vi "Parse qUSG CMD Answer.vi"(0 "Answer To Parse":string, 5 "error in":errorcluster) -> (14 "Array of CommandInfo":T1[](array[typedef]), 19 "error out":errorcluster)   [LabVIEW 2020]
doc: "Parse a SPV? structured answer to a array of parameter sets.\nWill return a warning if some parameters could not be parsed."
uses:
  General command.llb/CommandInfo.ctl
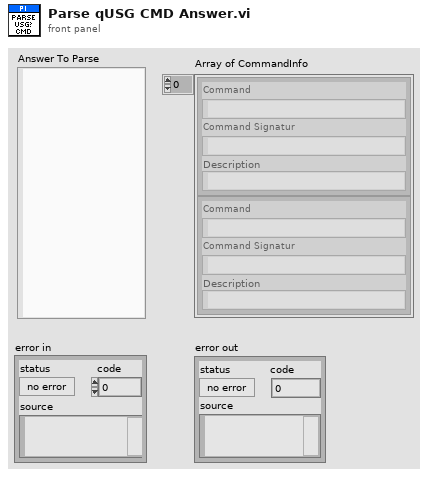
[diagram p1: front panel]
types:
  T1 = typedef "CommandInfo.ctl" = cluster{"Command":string, "Command Signatur":string, "Description":string}
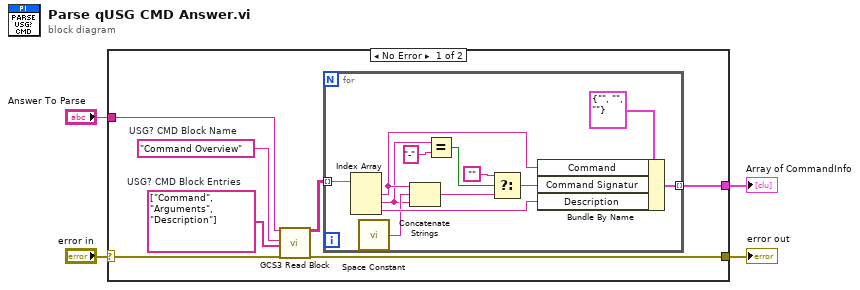
[diagram p0: block diagram]
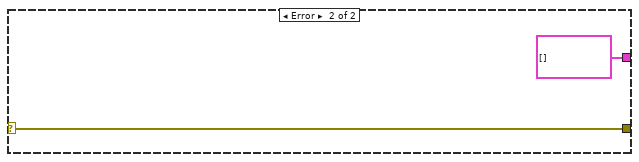
[diagram p2: hidden frame]
diagram:
  n1 = case shown="No Error" "error in" {
    selector: "error in" -> [w10 w25]
    tunnel: "Answer To Parse" -> [w11 _]
    tunnel: [w5 T1[] []] -> w1
    tunnel: [w6 w25] -> w2
    frame No Error {
      w7 = string[] ["Command", "Arguments", "Description"]  # USG? CMD Block Entries
      w8 = "Command Overview"  # USG? CMD Block Name
      n2 = call "GCS3 Read Block.vi"("GCS 3.0 Block to Parse"=w11, "Expected GCS 3.0 Block Name"=w8, "List of expected GCS 3.0 Block Entries"=w7, "error in"=w10) -> ("List of extracted GCS 3.0 Block Entries"=w9:string[][], "error out"=w6:errorcluster)  [unwired: 14 in]
      n3 = for {
        tunnel: w9 -> [w20] mode=indexing
        tunnel: [w21] -> w5 mode=indexing
        n4 = Index Array(array=w20) -> (element #1=w14:string, element #2=w13:string, element #3=w23:string)  [unwired: 3 in]
        n5 = call <vilib>:"Space Constant.vi"() -> ("String"=w15:string)
        n6 = Concatenate Strings(w14, w15, w13) -> (w16:string)
        n7 = Equal?(x=w13, y="-") -> (x = y?=w19:bool)
        n8 = Select(t="", s=w19, f=w16) -> (s? t:f=w12:string)
        n9 = Bundle By Name(cluster=T1 {"Command"="", "Command Signatur"="", "Description"=""} ("CommandInfo"), "Command"=w14, "Command Signatur"=w12, "Description"=w23) -> (w21:T1)
      }
    }
    frame Error {
    }
  }
  "error out" <- w2
  "Array of CommandInfo" <- w1
